vi "tcp_send_and_receive_working.vi"() -> ()   [LabVIEW 2021]
panel:
  out "data out":string
  in  "stop 2":bool
  in  "stop":bool
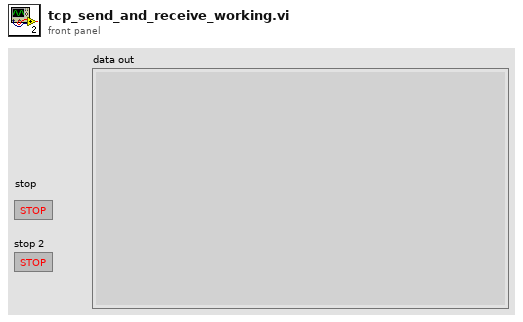
[diagram p1: front panel]
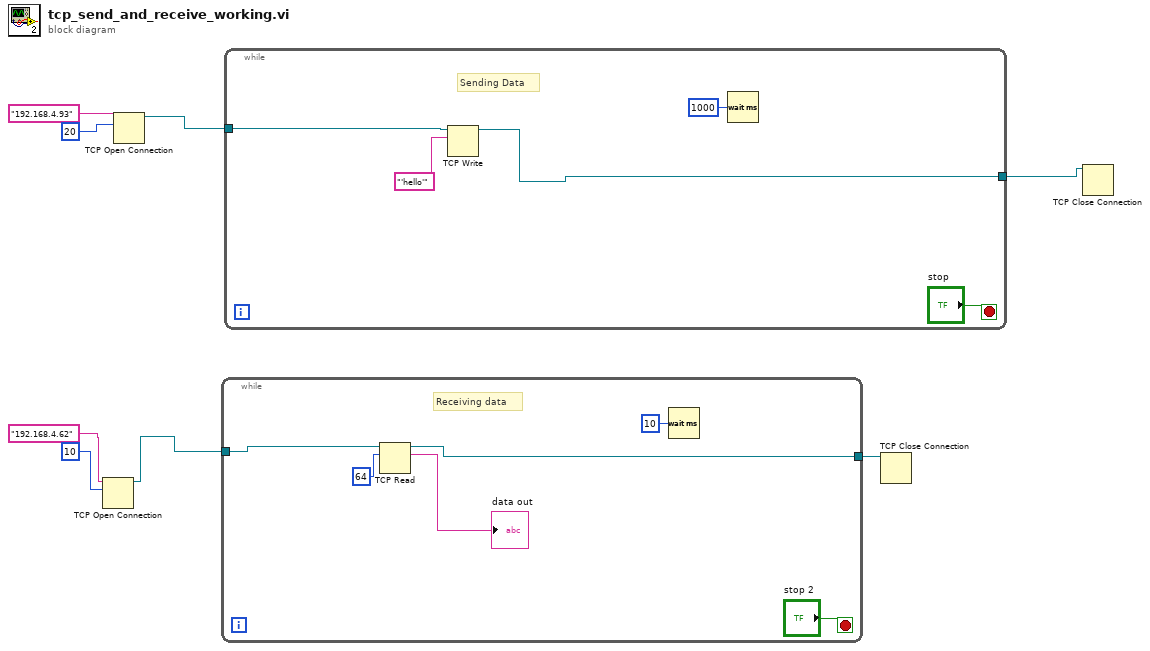
[diagram p0: block diagram]
diagram:
  n1 = TCP Open Connection(address="192.168.4.62", remote port or service name=u16 10) -> (connection ID=w2:refnum<k5>)  [unwired: 3 in, 1 out]
  n2 = TCP Open Connection(address="192.168.4.93", remote port or service name=u16 20) -> (connection ID=w5:refnum<k5>)  [unwired: 3 in, 1 out]
  n3 = while {
    tunnel: w2 -> [w12]
    tunnel: [w11] -> w4
    stop <- "stop 2" stop-if-true
    # "Receiving data"
    n4 = TCP Read(connection ID=w12, bytes to read=64) -> (connection ID out=w11:refnum<k5>, data out=→"data out":string)  [unwired: 3 in, 1 out]
    n5 = Wait (ms)(milliseconds to wait=u32 10) -> ()  [unwired: 1 out]
  }
  n6 = while {
    tunnel: [w17] -> w8
    tunnel: w5 -> [w16]
    stop <- "stop" stop-if-true
    # "Sending Data"
    n7 = TCP Write(connection ID=w16, data in="'hello'") -> (connection ID out=w17:refnum<k5>)  [unwired: 2 in, 2 out]
    n8 = Wait (ms)(milliseconds to wait=u32 1000) -> ()  [unwired: 1 out]
  }
  n9 = TCP Close Connection(connection ID=w4) -> ()  [unwired: 2 in, 2 out]
  n10 = TCP Close Connection(connection ID=w8) -> ()  [unwired: 2 in, 2 out]
